vi "Enqueue Write.vi"(5 "Timeout":i32, 6 "Data":string, 7 "Response":bool, 8 "error in (no error)":errorcluster, 9 "Function ID":u8, 10 "Stack ID":u8, 11 "Write":refnum<queue>) -> (0 "error out":errorcluster, 3 "GUID":string)   [LabVIEW 2011, in "Tinkerforge.lvlib" / "IP Connection.lvclass"]
doc: "This VI enqueues a write command to the write queue."
uses:
  IP Connection.lvclass
  Type Definitions/Message.ctl
  Tinkerforge.lvlib
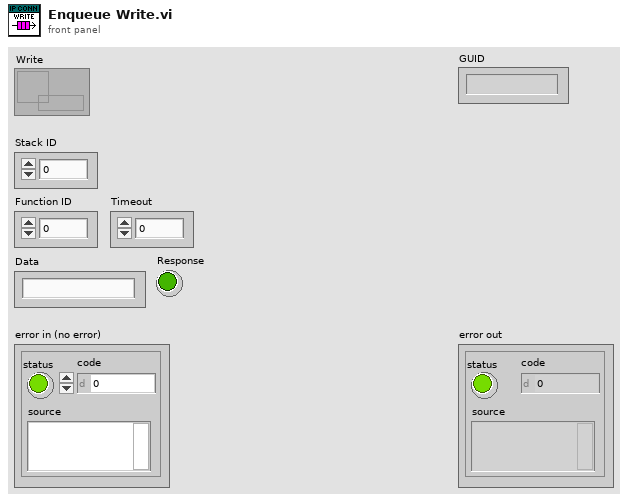
[diagram p1: front panel]
types:
  T1 = typedef "Tinkerforge.lvlib/IP Connection.lvclass/Message.ctl" = cluster{"Stack ID":u8, "Function ID":u8, "Data":string, "Request GUID":string, "Timeout":i32, "Response":bool}
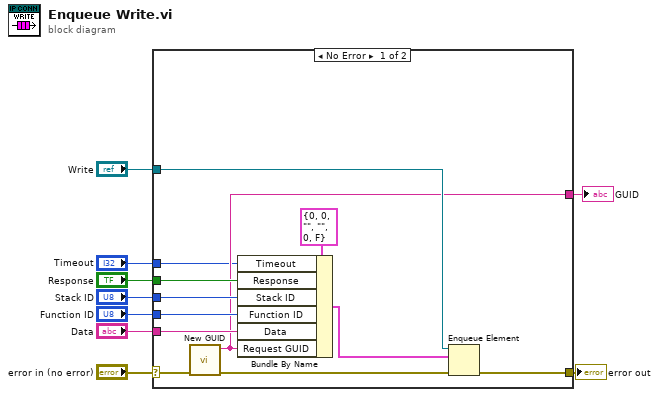
[diagram p0: block diagram]
diagram:
  n1 = case shown="No Error" "error in (no error)" {
    selector: "error in (no error)" -> [w15 w22]
    tunnel: [w21 w22] -> w8
    tunnel: "Data" -> [w18 _]
    tunnel: "Function ID" -> [w17 _]
    tunnel: "Stack ID" -> [w16 _]
    tunnel: "Response" -> [w13 _]
    tunnel: "Write" -> [w12 _]
    tunnel: [w11 _] -> w2
    tunnel: "Timeout" -> [w10 _]
    frame No Error {
      n2 = call "New GUID.vi"("Error In"=w15) -> ("Error Out"=w14:errorcluster, "GUID"=w11:string)  [unwired: 9 in]
      n3 = Bundle By Name(cluster=T1 {"Stack ID"=0, "Function ID"=0, "Data"="", "Request GUID"="", "Timeout"=0, "Response"=FALSE} ("element"), "Timeout"=w10, "Response"=w13, "Stack ID"=w16, "Function ID"=w17, "Data"=w18, "Request GUID"=w11) -> (w19:T1)
      n4 = Enqueue Element(queue=w12, element=w19, error in (no error)=w14) -> (error out=w21:errorcluster)  [unwired: 1 in, 2 out]
    }
    frame Error {
    }
  }
  "error out" <- w8
  "GUID" <- w2
